vi "Load Config.vi"(8 "Error In":errorcluster, 11 "Config File Path Override":path) -> (0 "Error Out":errorcluster, 3 "VIChallenge Config":T1)   [LabVIEW 2013, in "VIChallenge.lvlib"]
uses:
  VIChallenge.lvlib
  Type Defs/VIChallenge Config.ctl
  <vilib>/National Instruments/NI Amazon Web Services (AWS) Toolkit for LabVIEW/SQS/VI Source/AWS SQS Class/AWS_SQS.lvclass
  <vilib>/National Instruments/NI Amazon Web Services (AWS) Toolkit for LabVIEW/AWS Core Lib/VI Source/Canonicals/AWS_Core Canonical Credentials/Canonical Credentials.lvclass
  <vilib>/National Instruments/NI Amazon Web Services (AWS) Toolkit for LabVIEW/AWS Core Lib/VI Source/Canonicals/AWS_Core Canonical Required Parameters/Canonical Required Parameters.lvclass
  <vilib>/National Instruments/NI Amazon Web Services (AWS) Toolkit for LabVIEW/SQS/VI Source/Canonicals/Canonical CreateQueue/Canonical CreateQueue.lvclass
  <vilib>/National Instruments/NI Amazon Web Services (AWS) Toolkit for LabVIEW/SQS/VI Source/Canonicals/Canonical ListQueues/Canonical ListQueues.lvclass
  <vilib>/National Instruments/NI Amazon Web Services (AWS) Toolkit for LabVIEW/SQS/VI Source/Canonicals/Canonical AddPermission/Canonical AddPermission.lvclass
  <vilib>/National Instruments/NI Amazon Web Services (AWS) Toolkit for LabVIEW/SQS/VI Source/Canonicals/Canonical ChangeMessageVisibility/Canonical ChangeMessageVisibility.lvclass
  <vilib>/National Instruments/NI Amazon Web Services (AWS) Toolkit for LabVIEW/SQS/VI Source/Canonicals/Canonical ChangeMessageVisibilityBatch/Canonical ChangeMessageVisibilityBatch.lvclass
  <vilib>/National Instruments/NI Amazon Web Services (AWS) Toolkit for LabVIEW/SQS/VI Source/Canonicals/Canonical DeleteMessage/Canonical DeleteMessage.lvclass
  <vilib>/National Instruments/NI Amazon Web Services (AWS) Toolkit for LabVIEW/SQS/VI Source/Canonicals/Canonical DeleteMessageBatch/Canonical DeleteMessageBatch.lvclass
  <vilib>/National Instruments/NI Amazon Web Services (AWS) Toolkit for LabVIEW/SQS/VI Source/Canonicals/Canonical GetQueueAttributes/Canonical GetQueueAttributes.lvclass
  <vilib>/National Instruments/NI Amazon Web Services (AWS) Toolkit for LabVIEW/SQS/VI Source/Canonicals/Canonical GetQueueUrl/Canonical GetQueueUrl.lvclass
  <vilib>/National Instruments/NI Amazon Web Services (AWS) Toolkit for LabVIEW/SQS/VI Source/Canonicals/Canonical ReceiveMessage/Canonical ReceiveMessage.lvclass
  <vilib>/National Instruments/NI Amazon Web Services (AWS) Toolkit for LabVIEW/SQS/VI Source/Canonicals/Canonical RemovePermission/Canonical RemovePermission.lvclass
  <vilib>/National Instruments/NI Amazon Web Services (AWS) Toolkit for LabVIEW/SQS/VI Source/Canonicals/Canonical SendMessage/Canonical SendMessage.lvclass
  <vilib>/National Instruments/NI Amazon Web Services (AWS) Toolkit for LabVIEW/SQS/VI Source/Canonicals/Canonical SendMessageBatch/Canonical SendMessageBatch.lvclass
  <vilib>/National Instruments/NI Amazon Web Services (AWS) Toolkit for LabVIEW/SQS/VI Source/Canonicals/Canonical SetQueueAttributes/Canonical SetQueueAttributes.lvclass
  <vilib>/National Instruments/NI Amazon Web Services (AWS) Toolkit for LabVIEW/AWS Core Lib/VI Source/Typedefs/AWS_AWS Credentials.ctl
  Type Defs/JSON_job.ctl
  <vilib>/addons/database/Connection.llb/Conn ObjectReference.ctl
  Grader/Type Defs/Challenge.ctl
  <vilib>/National Instruments/NI Amazon Web Services (AWS) Toolkit for LabVIEW/SQS/VI Source/Public Typedefs/AWS_SQS Queue Name and Account Number.ctl
  <vilib>/Utility/config.llb/Read Key (String).vi
  <vilib>/Utility/config.llb/Read Key (Path).vi
  <vilib>/Utility/config.llb/NI_LVConfig.lvlib
  <vilib>/National Instruments/NI Amazon Web Services (AWS) Toolkit for LabVIEW/AWS Core Lib/VI Source/AWS_Core.lvlib
  <vilib>/National Instruments/NI Amazon Web Services (AWS) Toolkit for LabVIEW/SQS/VI Source/AWS_SQS.lvlib
  <vilib>/National Instruments/LabVIEW Interface for Amazon S3/LV Interface for Amazon S3.lvlib
  <vilib>/addons/database/NI_Database_API.lvlib
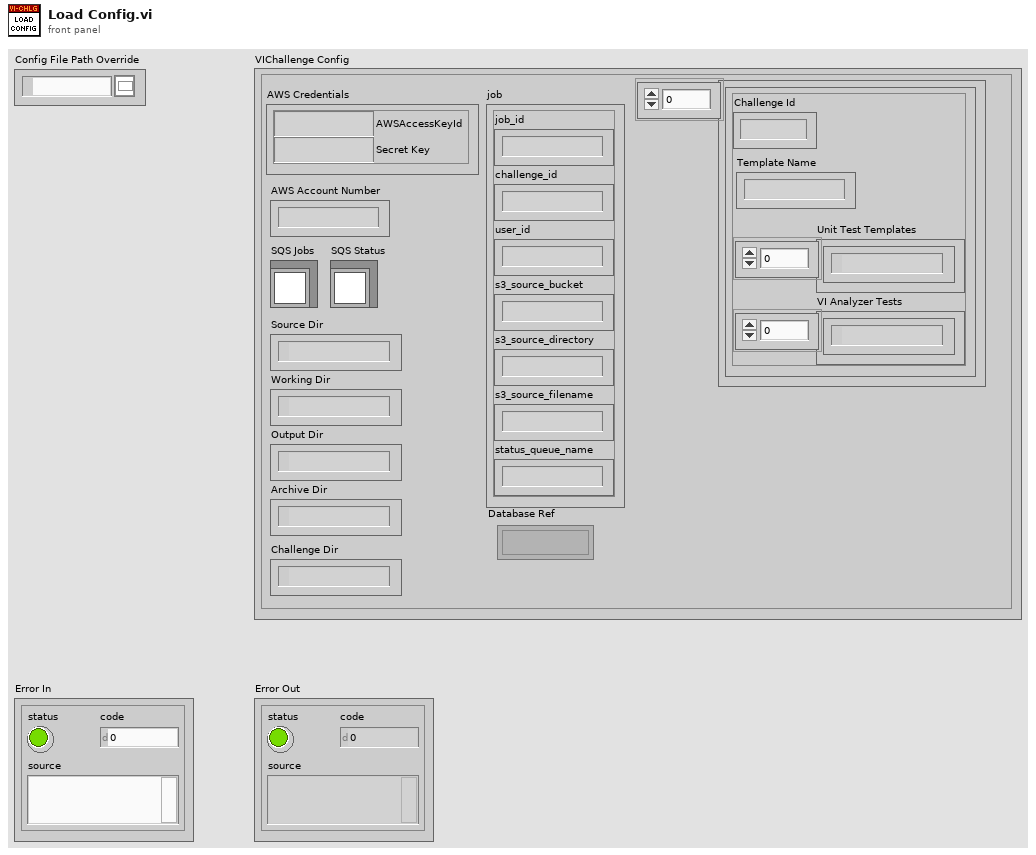
[diagram p1: front panel]
types:
  T1 = typedef "VIChallenge.lvlib/VIChallenge Config.ctl" = cluster{"AWS Credentials":T2, "AWS Account Number":string, "SQS Jobs":refnum<class "AWS_SQS.lvclass">, "SQS Status":refnum<class "AWS_SQS.lvclass">, "Source Dir":path, "Working Dir":path, "Output Dir":path, "Archive Dir":path, "job":T3, "Database Ref":T4, "Challenge Dir":path, "Challenges":T5[]}
  T2 = typedef "AWS_Core.lvlib/AWS_AWS Credentials.ctl" = cluster{"AWSAccessKeyId":string, "Secret Key":string}
  T3 = typedef "VIChallenge.lvlib/JSON_job.ctl" = cluster{"job_id":string, "challenge_id":string, "user_id":string, "s3_source_bucket":string, "s3_source_directory":string, "s3_source_filename":string, "status_queue_name":string}
  T4 = typedef "NI_Database_API.lvlib/Conn ObjectReference.ctl" = refnum<k1>
  T5 = typedef "VIChallenge.lvlib/Challenge.ctl" = cluster{"Challenge Id":i32, "Unit Test Templates":path[], "VI Analyzer Tests":path[], "Template Name":string}
  T6 = typedef "AWS_SQS.lvlib/AWS_SQS Queue Name and Account Number.ctl" = cluster{"QueueName":string, "Account Number":string}
  T7 = typedef "NI_LVConfig.lvlib/Config Data RefNum.ctl" = refnum<k1>
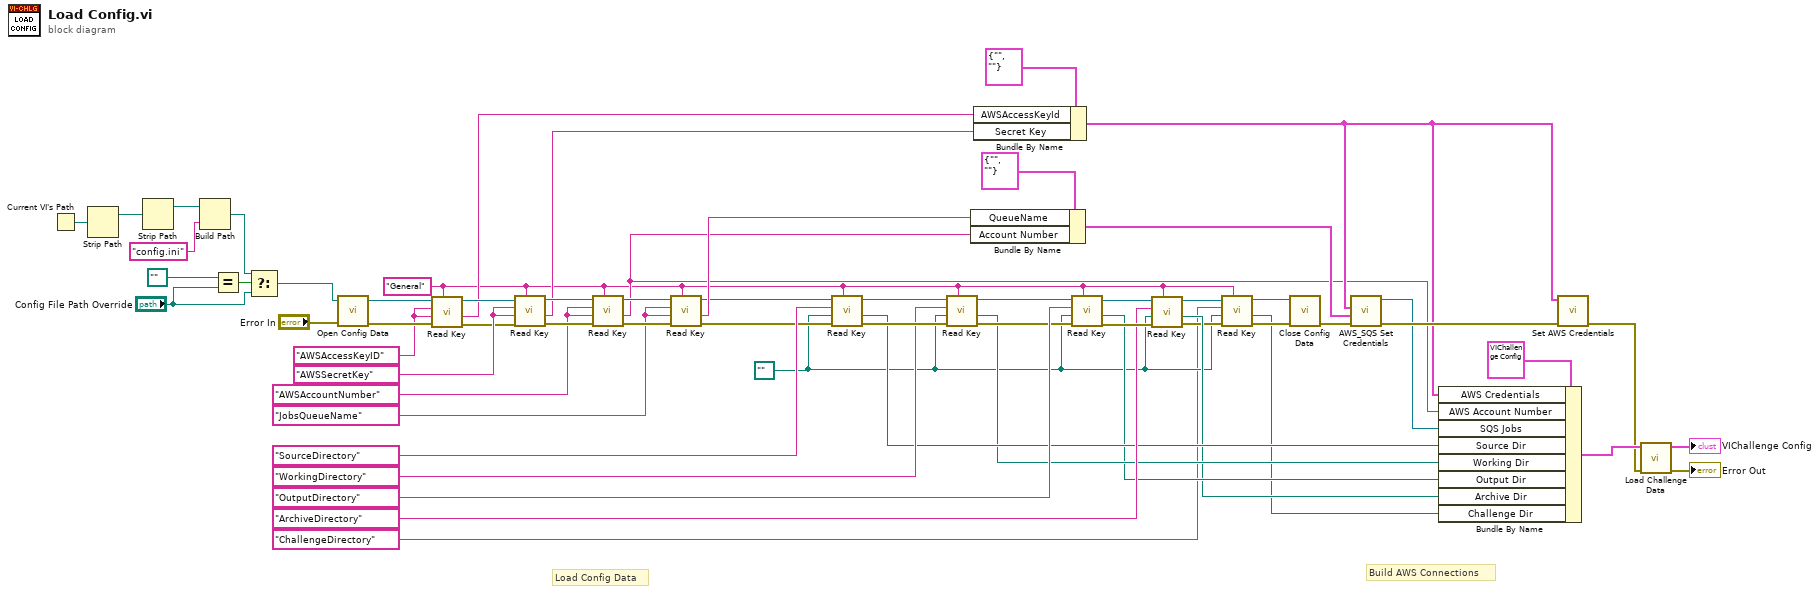
[diagram p0: block diagram]
diagram:
  w2 = path "" ("Unzip Directory")
  w55 = "JobsQueueName"
  w56 = "AWSAccountNumber"
  w57 = "AWSSecretKey"
  w58 = "AWSAccessKeyID"
  w4 = "General" ("section")
  # "Build AWS Connections"
  # "Load Config Data"
  n1 = Current VI's Path() -> (path=w45:path)
  n2 = Strip Path(path=w45) -> (stripped path=w44:path)  [unwired: 1 out]
  n3 = Strip Path(path=w44) -> (stripped path=w43:path)  [unwired: 1 out]
  n4 = Build Path(base path=w43, name or relative path="config.ini") -> (appended path=w10:path)
  n5 = Equal?(x=path "", y="Config File Path Override") -> (x = y?=w13:bool)
  n6 = Select(t=w10, s=w13, f="Config File Path Override") -> (s? t:f=w12:path)
  n7 = call <vilib>:"Open Config Data.vi"("error in (no error)"="Error In", "configuration file path"=w12) -> ("error out"=w62:errorcluster, "refnum"=w48:T7)  [unwired: 7 in, 1 out]
  n8 = call-poly <vilib>:"Read Key.vi"("section"=w4, "error in (no error)"=w62, "default value"=w58, "key"=w58, "refnum"=w48) -> ("error out"=w49:errorcluster, "value"=w40:string, "refnum out"=w47:T7)  [unwired: 3 in, 1 out]
  n9 = call-poly <vilib>:"Read Key.vi"("section"=w4, "error in (no error)"=w49, "default value"=w57, "key"=w57, "refnum"=w47) -> ("error out"=w61:errorcluster, "value"=w39:string, "refnum out"=w52:T7)  [unwired: 3 in, 1 out]
  n10 = call-poly <vilib>:"Read Key.vi"("section"=w4, "error in (no error)"=w61, "default value"=w56, "key"=w56, "refnum"=w52) -> ("error out"=w60:errorcluster, "value"=w18:string, "refnum out"=w51:T7)  [unwired: 3 in, 1 out]
  n11 = call-poly <vilib>:"Read Key.vi"("section"=w4, "error in (no error)"=w60, "default value"=w55, "key"=w55, "refnum"=w51) -> ("error out"=w27:errorcluster, "value"=w37:string, "refnum out"=w26:T7)  [unwired: 3 in, 1 out]
  n12 = call-poly <vilib>:"Read Key.vi"("section"=w4, "error in (no error)"=w27, "default value"=w2, "key"="SourceDirectory", "refnum"=w26) -> ("error out"=w59:errorcluster, "value"=w25:path, "refnum out"=w50:T7)  [unwired: 3 in, 1 out]
  n13 = call-poly <vilib>:"Read Key.vi"("section"=w4, "error in (no error)"=w59, "default value"=w2, "key"="WorkingDirectory", "refnum"=w50) -> ("error out"=w30:errorcluster, "value"=w24:path, "refnum out"=w29:T7)  [unwired: 3 in, 1 out]
  n14 = Bundle By Name(cluster=T6 {"QueueName"="", "Account Number"=""} ("Queue Name and Account Number"), "QueueName"=w37, "Account Number"=w18) -> (w36:T6)
  n15 = Bundle By Name(cluster=T2 {"AWSAccessKeyId"="", "Secret Key"=""} ("AWS Credentials"), "AWSAccessKeyId"=w40, "Secret Key"=w39) -> (w19:T2)
  n16 = call-poly <vilib>:"Read Key.vi"("section"=w4, "error in (no error)"=w30, "default value"=w2, "key"="OutputDirectory", "refnum"=w29) -> ("error out"=w32:errorcluster, "value"=w23:path, "refnum out"=w33:T7)  [unwired: 3 in, 1 out]
  n17 = call-poly <vilib>:"Read Key.vi"("section"=w4, "error in (no error)"=w32, "default value"=w2, "key"="ArchiveDirectory", "refnum"=w33) -> ("error out"=w7:errorcluster, "value"=w22:path, "refnum out"=w6:T7)  [unwired: 3 in, 1 out]
  n18 = call-poly <vilib>:"Read Key.vi"("section"=w4, "error in (no error)"=w7, "default value"=w2, "key"="ChallengeDirectory", "refnum"=w6) -> ("error out"=w8:errorcluster, "value"=w3:path, "refnum out"=w5:T7)  [unwired: 3 in, 1 out]
  n19 = call <vilib>:"Close Config Data.vi"("error in (no error)"=w8, "refnum"=w5) -> ("error out"=w21:errorcluster)  [unwired: 8 in, 1 out]
  n20 = call <vilib>:"AWS_SQS Set Credentials.vi"("error in (no error)"=w21, "Queue Name and Account Number"=w36, "AWS Credentials"=w19) -> ("error out"=w35:errorcluster, "AWS_SQS out"=w20:refnum<class "AWS_SQS.lvclass">)  [unwired: 7 in]
  n21 = Bundle By Name(cluster=T1 {"AWS Credentials"={"AWSAccessKeyId"="", "Secret Key"=""}, "AWS Account Number"="", "SQS Jobs"=refnum, "SQS Status"=refnum, "Source Dir"=path "", "Working Dir"=path "", "Output Dir"=path "", "Archive Dir"=path "", "job"={"job_id"="", "challenge_id"="", "user_id"="", "s3_source_bucket"="", "s3_source_directory"="", "s3_source_filename"="", "status_queue_name"=""}, "Database Ref"=refnum, "Challenge Dir"=path "", "Challenges"=[]} ("VIChallenge Config"), "AWS Credentials"=w19, "AWS Account Number"=w18, "SQS Jobs"=w20, "Source Dir"=w25, "Working Dir"=w24, "Output Dir"=w23, "Archive Dir"=w22, "Challenge Dir"=w3) -> (w17:T1)
  n22 = call <vilib>:"Set AWS Credentials.vi"("error in (no error)"=w35, "AWS Credentials in"=w19) -> ("error out"=w16:errorcluster)  [unwired: 9 in]
  n23 = call "Load Challenge Data.vi"("Error In"=w16, "VIChallenge Config"=w17) -> ("Error Out"=→"Error Out":errorcluster, "VIChallenge Config"=→"VIChallenge Config":T1)  [unwired: 7 in, 1 out]
